vi "cw_5_6.vi"() -> ()   [LabVIEW 2022 SP3]
panel:
  out "XY Graph":cluster{i32[], u32[]}[](graph)
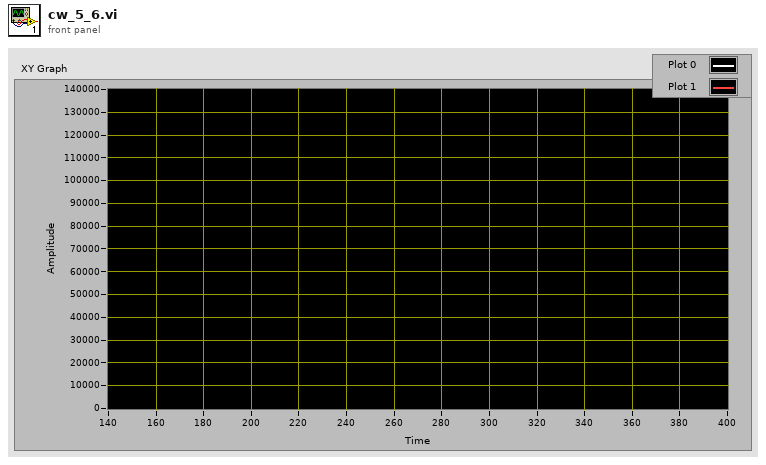
[diagram p1: front panel]
types:
  T1 = enum16{"big-endian, network order", "native, host order", "little-endian"}
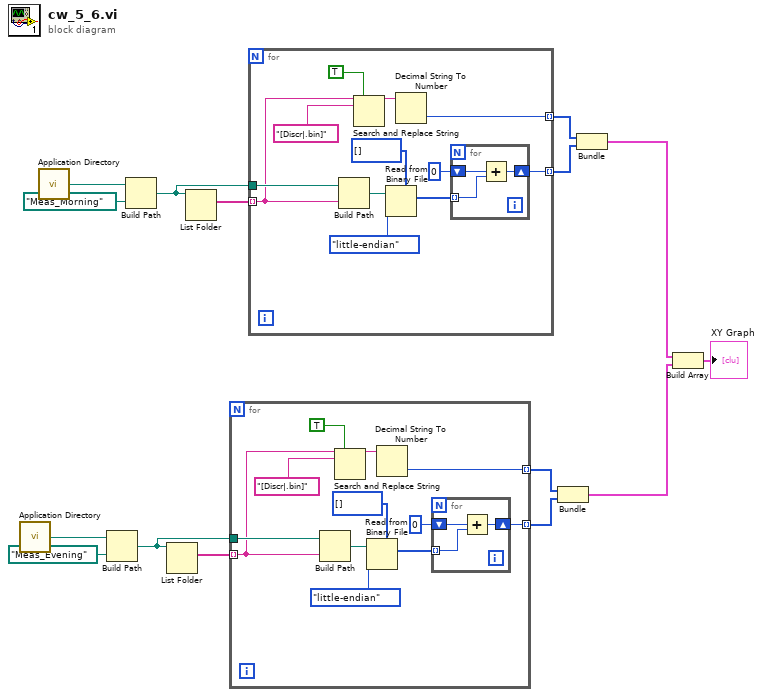
[diagram p0: block diagram]
diagram:
  n1 = call <vilib>:"Application Directory.vi"() -> ("Application Directory"=w9:path)
  n2 = call <vilib>:"Application Directory.vi"() -> ("Application Directory"=w15:path)
  n3 = Build Path(base path=w9, name or relative path=path "Meas_Evening") -> (appended path=w6:path)
  n4 = Build Path(base path=w15, name or relative path=path "Meas_Morning") -> (appended path=w12:path)
  n5 = List Folder(path=w6) -> (filenames=w7:string[])  [unwired: 3 in, 3 out]
  n6 = List Folder(path=w12) -> (filenames=w13:string[])  [unwired: 3 in, 3 out]
  n7 = for {
    tunnel: w7 -> [w19] mode=indexing
    tunnel: w6 -> [w27]
    tunnel: [w17] -> w5 mode=indexing
    tunnel: [w16] -> w4 mode=indexing
    n8 = Build Path(base path=w27, name or relative path=w19) -> (appended path=w26:path)
    n9 = Search and Replace String(replace all?=TRUE ("replace all? (F)"), input string=w19, search string="[Discr|.bin]") -> (result string=w18:string)  [unwired: 5 in, 3 out]
    n10 = Read from Binary File(5:u32[] [], 9:T1."little-endian" ("byte order (0:big-endian, network order)"), 11:w26) -> (2:w23:u32[])  [unwired: 3 in, 3 out]
    n11 = Decimal String To Number(string=w18) -> (number=w17:i32)  [unwired: 2 in, 1 out]
    n12 = for {
      tunnel: w23 -> [w29] mode=indexing
      shift-right: [w28] -> w16
      shift-left: u32 0 -> [w30]
      n13 = Add(x=w30, y=w29) -> (x+y=w28:u32)
    }
  }
  n14 = for {
    tunnel: w13 -> [w34] mode=indexing
    tunnel: w12 -> [w42]
    tunnel: [w32] -> w11 mode=indexing
    tunnel: [w31] -> w10 mode=indexing
    n15 = Build Path(base path=w42, name or relative path=w34) -> (appended path=w41:path)
    n16 = Search and Replace String(replace all?=TRUE ("replace all? (F)"), input string=w34, search string="[Discr|.bin]") -> (result string=w33:string)  [unwired: 5 in, 3 out]
    n17 = Read from Binary File(5:u32[] [], 9:T1."little-endian" ("byte order (0:big-endian, network order)"), 11:w41) -> (2:w38:u32[])  [unwired: 3 in, 3 out]
    n18 = Decimal String To Number(string=w33) -> (number=w32:i32)  [unwired: 2 in, 1 out]
    n19 = for {
      tunnel: w38 -> [w44] mode=indexing
      shift-right: [w43] -> w31
      shift-left: u32 0 -> [w45]
      n20 = Add(x=w45, y=w44) -> (x+y=w43:u32)
    }
  }
  n21 = Bundle(w5, w4) -> (w2:cluster{i32[], u32[]})  [unwired: 1 in]
  n22 = Bundle(w11, w10) -> (w3:cluster{i32[], u32[]})  [unwired: 1 in]
  n23 = Build Array(w3, w2) -> (→"XY Graph":cluster{i32[], u32[]}[])
